vi "oneorminusone.vi"(10 "input 2":dbl[](array[numeric]), 11 "input1":dbl[](array[numeric])) -> (2 "output2":i32[](array[numeric]), 3 "output1":i32[](array[numeric]))   [LabVIEW 2014]
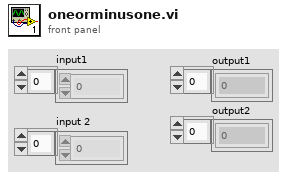
[diagram p1: front panel]
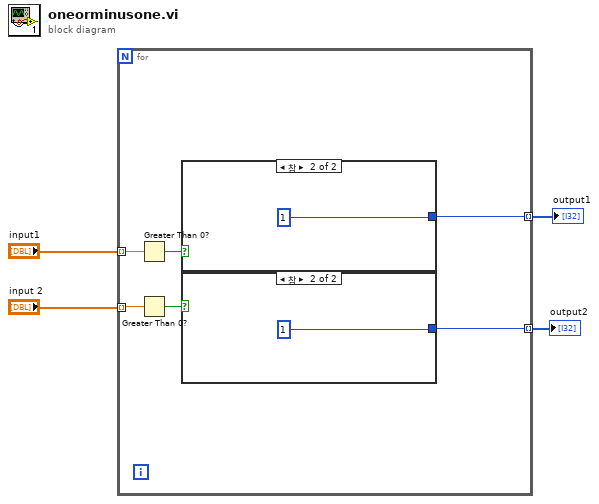
[diagram p0: block diagram]
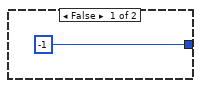
[diagram p2: hidden frame]
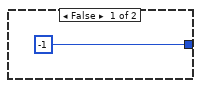
[diagram p3: hidden frame]
diagram:
  n1 = for {
    tunnel: "input1" -> [w10] mode=indexing
    tunnel: "input 2" -> [w7] mode=indexing
    tunnel: [w6] -> w2 mode=indexing
    tunnel: [w5] -> w1 mode=indexing
    n2 = Greater Than 0?(x=w10) -> (x > 0?=w9:bool)
    n3 = Greater Than 0?(x=w7) -> (x > 0?=w8:bool)
    n4 = case shown="참" w9 {
      tunnel: [-1 1] -> w6
      frame False {
      }
      frame True {
      }
    }
    n5 = case shown="참" w8 {
      tunnel: [-1 1] -> w5
      frame False {
      }
      frame True {
      }
    }
  }
  "output1" <- w2
  "output2" <- w1
